vi "8.8.1.vi"() -> ()   [LabVIEW 2018]
panel:
  out "b":dbl(graph)
  in  "정지":bool
  out "a":dbl(graph)
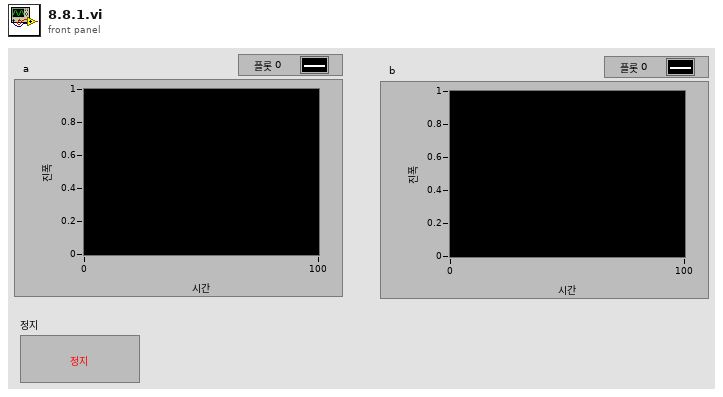
[diagram p1: front panel]
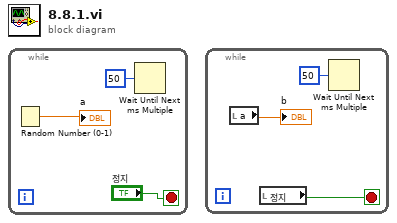
[diagram p0: block diagram]
diagram:
  n1 = while {
    stop <- "정지" stop-if-true
    n2 = Random Number (0-1)() -> (number: 0 to 1=→"a":dbl)
    n3 = Wait Until Next ms Multiple(millisecond multiple=u32 50 ("ms 배수")) -> ()  [unwired: 1 out]
  }
  n4 = while {
    stop <- w4 stop-if-true
    n5 = local read "a"() -> (→"b":dbl)
    n6 = local read "정지"() -> (w4:bool)
    n7 = Wait Until Next ms Multiple(millisecond multiple=u32 50 ("ms 배수")) -> ()  [unwired: 1 out]
  }
